vi "Initialize.vi"(8 "error in":errorcluster, 10 "parameters":variant, 11 "node in":refnum<class "TimingSource.lvclass">) -> (0 "error out":errorcluster, 2 "summary":T2[](array[typedef]), 3 "data value reference":T1)   [LabVIEW 2019, in "TimingSource.lvclass"]
doc: "Initializes the data of a node to its default state.\nThe object is not created inside of this VI, because it is created from a File depending on user selection.\nCopyright 2015 National Instruments Corporation\n\nLicensed under the Apache License, Version 2.0 (the \"License\"); you may not use this file except in compliance with the License. You may obtain a copy of the License at http://www.apache.org/licenses/LICENSE-2.0\nUnless required by applicable law or agreed to in writing, software distributed under the License is distributed on an \"AS IS\" BASIS, WITHOUT WARRANTIES OR CONDITIONS OF ANY KIND, either express or implied. See the License for the specific language governing permissions and limitations under the License."
uses:
  TimingSource.lvclass
  C:/Program Files (x86)/National Instruments/LabVIEW 2019/vi.lib/NI/Configuration Framework/Node/NISE_CEF_Node.lvclass
  <vilib>/NI/Configuration Framework/Node/Summary.ctl
  <vilib>/NI/Configuration Framework/Node/NodeRef.ctl
  <vilib>/NI/Configuration Framework/Node/NISE_CEF_Node.lvclass
  XML Controls/Timing Source Properties.ctl
  XML Controls/Timing Source Source Distribution Properties.ctl
  XML Controls/Supported Targets.ctl
  XML Controls/Path Cluster.ctl
  <vilib>/NI/Configuration Framework/Node/NISE_CEF_Node.lvclass/NISE_CEF_Node.ctl
  Target/Target.lvclass
  Target/Target.lvclass/Target.ctl
  TimingSource.lvclass/TimingSource.ctl
  Target/Read Source.vi
  <vilib>/NI/Configuration Framework/Node/ReadParent.vi
  <vilib>/NI/Configuration Framework/Node/ReadChildren.vi
  Write Timing Source Properties.vi
  <vilib>/NI/Configuration Framework/Node/ReadNodeClass.vi
  VeriStand Custom Device XML Parser.lvlib
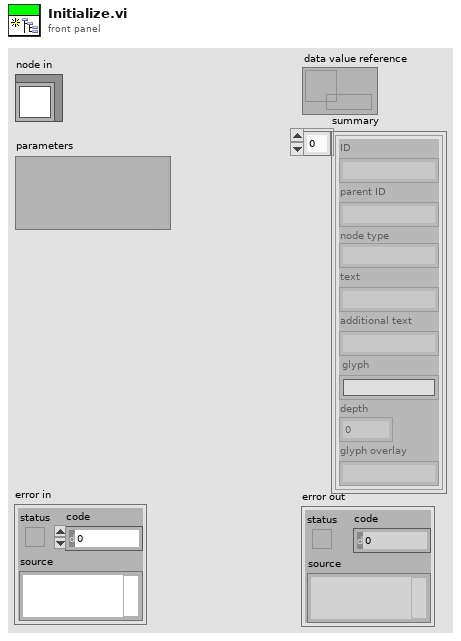
[diagram p1: front panel]
types:
  T1 = typedef "NISE_CEF_Node.lvclass/NodeRef.ctl" = refnum<data-value>
  T2 = typedef "NISE_CEF_Node.lvclass/Summary.ctl" = cluster{"ID":string, "parent ID":string, "node type":string, "text":string, "additional text":string, "glyph":string, "depth":i32, "glyph overlay":string}
  T3 = typedef "VeriStand Custom Device XML Parser.lvlib/Timing Source Properties.ctl" = cluster{"Has Timing Source Capability":bool, "Source Distribution":T4}
  T4 = typedef "VeriStand Custom Device XML Parser.lvlib/Timing Source Source Distribution Properties.ctl" = cluster{"Supported Target":T5, "Source":T6, "Real Time System Destination":string, "Version":string}[]
  T5 = typedef "VeriStand Custom Device XML Parser.lvlib/Supported Targets.ctl" = enum16{"All", "Pharlap", "VxWorks", "Windows", "Linux_32_ARM", "Linux_x64", "PharlapWindows", "PharlapVxWorks", "VxWorksWindows"}
  T6 = typedef "VeriStand Custom Device XML Parser.lvlib/Path Cluster.ctl" = cluster{"Path":path, "Path Type":enum16{"Absolute", "To Base", "To Common Doc Dir", "To Application Data Dir"}}
  T7 = cluster{"Supported Target":T5, "Source":T6, "Real Time System Destination":string, "Version":string}
  T8 = typedef "VeriStand XML Parser.lvlib/Path Cluster.ctl" = cluster{"Path":path, "Path Type":enum16{"Absolute", "To Base", "To Common Doc Dir", "To Application Data Dir"}}
  T9 = typedef "VeriStand XML Parser.lvlib/Supported Targets.ctl" = enum16{"All", "Pharlap", "VxWorks", "Windows", "Linux_32_ARM", "Linux_x64", "PharlapWindows", "PharlapVxWorks", "VxWorksWindows"}
  T10 = cluster{"Source":T8, "Real Time System Destination":string, "Supported Target":T9}
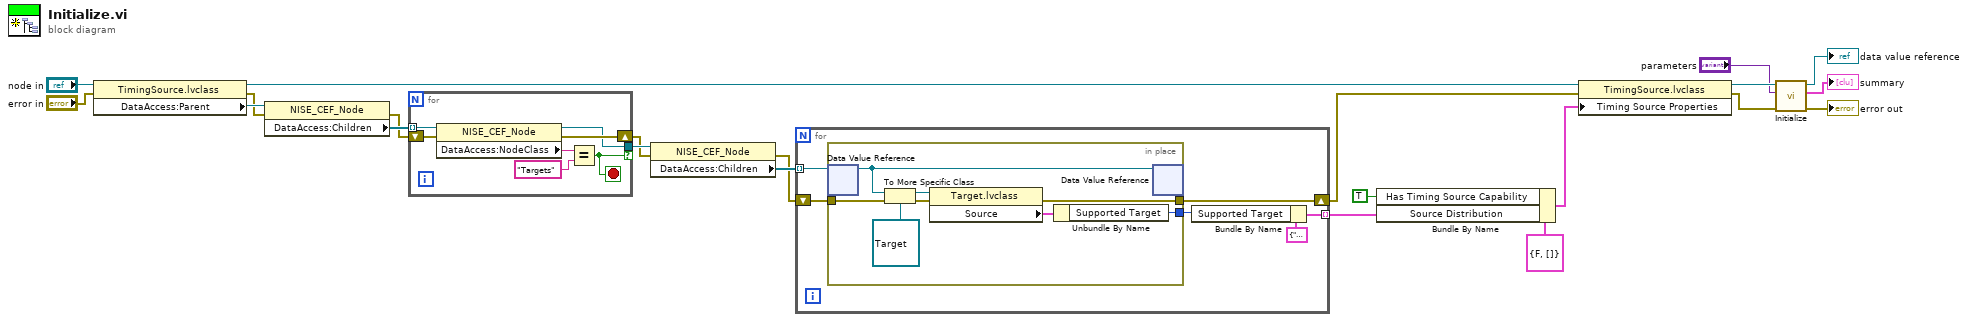
[diagram p0: block diagram]
diagram:
  n1 = property class="TimingSource.lvclass"(reference="node in", error in="error in") -> (reference out=w10:refnum<class "TimingSource.lvclass">, error out=w17:errorcluster, "DataAccess:Parent"=w18:T1)
  n2 = property class="NISE_CEF_Node"(reference=w18, error in=w17) -> (error out=w15:errorcluster, "DataAccess:Children"=w16:T1[])  [unwired: 1 out]
  n3 = for {
    tunnel: w16 -> [w29] mode=indexing
    shift-right: [w25] -> w13
    shift-left: w15 -> [w28]
    tunnel: [w24] -> w14 if=w23
    stop <- w23 stop-if-true
    n4 = property class="NISE_CEF_Node"(reference=w29, error in=w28) -> (reference out=w24:T1, error out=w25:errorcluster, "DataAccess:NodeClass"=w27:string)
    n5 = Equal?(x=w27, y="Targets" ("NodeClass")) -> (x = y?=w23:bool)
  }
  n6 = property class="NISE_CEF_Node"(reference=w14, error in=w13) -> (error out=w11:errorcluster, "DataAccess:Children"=w12:T1[])  [unwired: 1 out]
  n7 = for {
    tunnel: w12 -> [w35] mode=indexing
    shift-right: [w33] -> w5
    shift-left: w11 -> [w34]
    tunnel: [w30] -> w8 mode=indexing
    n8 = in-place {
      in-place-border: w34 -> [w43]
      in-place-border: [w37] -> w33
      in-place-border: [w36] -> w31
      n9 = in-place-dvr #1(w35) -> (w38:refnum<class "NISE_CEF_Node.lvclass">)  [unwired: 1 out]
      n10 = To More Specific Class(target class=refnum<class "Target.lvclass"> refnum ("Target.lvclass"), reference=w38, error in=w43) -> (specific class reference=w40:refnum<class "Target.lvclass">, error out=w41:errorcluster)
      n11 = property class="Target.lvclass"(reference=w40, error in=w41) -> (error out=w37:errorcluster, "Source"=w39:T10)  [unwired: 1 out]
      n12 = Unbundle By Name(w39) -> ("Supported Target"=w36:T9)
      n13 = in-place-dvr #1(w38) -> ()  [unwired: 2 out]
    }
    n14 = Bundle By Name(cluster=T7 {"Supported Target"=enum."All", "Source"={"Path"=path "", "Path Type"=enum."Absolute"}, "Real Time System Destination"="", "Version"=""} ("Source"), "Supported Target"=w31) -> (w30:T7)
  }
  n15 = Bundle By Name(cluster=T3 {"Has Timing Source Capability"=FALSE, "Source Distribution"=[]} ("Timing Source Properties"), "Has Timing Source Capability"=TRUE, "Source Distribution"=w8) -> (w6:T3)
  n16 = property class="TimingSource.lvclass"(reference=w10, error in=w5, "Timing Source Properties"=w6) -> (reference out=w3:refnum<class "TimingSource.lvclass">, error out=w2:errorcluster)
  n17 = call-parent "Initialize.vi"("error in"=w2, "parameters"="parameters", "node in"=w3) -> ("error out"=→"error out":errorcluster, "summary"=→"summary":T2[], "data value reference"=→"data value reference":T1)  [unwired: 6 in]
